vi "Camera.CaptureImage.vi"(8 "error in (no error)":errorcluster, 11 "Camera.Simulated":refnum<class "Camera.Simulated.lvclass">) -> (0 "error out":errorcluster, 2 "buffer":i32, 3 "Camera.Simulated out":refnum<class "Camera.Simulated.lvclass">)   [LabVIEW 2013, in "Camera.Simulated.lvclass"]
doc: "---------------------------------------------------------------\nJKI State Machine Objects™\nhttp://jki.net/state-machine-objects/\nCopyright (C) 2005-2015, JKI <info@jki.net>\nALL RIGHTS RESERVEDJKI State Machine Objects (SMO) 1.0.0.5\nJKI - JKI\nCopyright (c) 2016, JKI"
uses:
  Camera.Simulated.lvclass
  CircularBuffer/CircularBuffer.lvclass
  CircularBuffer.ImageData/CircularBuffer.ImageData.lvclass
  Camera/Camera.lvclass
panel:
  # "For instructions on how to use the JKI State Machine Objects, examples and video tutorials, visit:\nhttp://jki.net/state-machine-objects/\n\nJKI State Machine Objects™\nhttp://jki.net/state-machine-objects/\nCopyright (C) 2005-2015, JKI <info@jki.net>\nALL RIGHTS RESERVED"
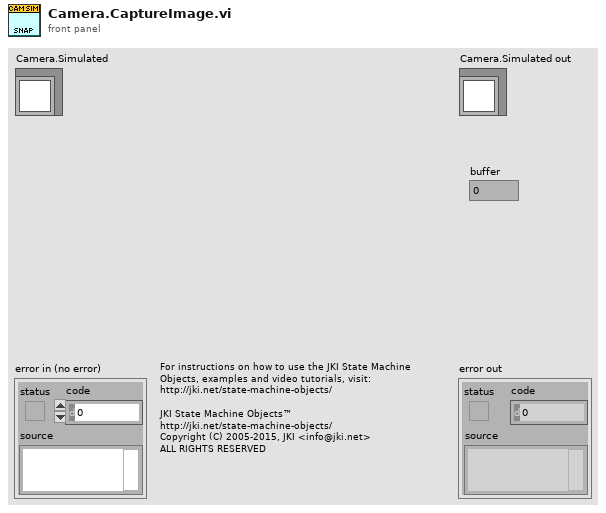
[diagram p1: front panel]
types:
  T1 = typedef "Camera.Simulated.lvclass/Dependencies--Cluster.ctl" = cluster{"CircularBuffer.ImageData":refnum<class "CircularBuffer.ImageData.lvclass">}
  T2 = typedef "imagedata.ctl" = cluster{"image type":i32, "image depth":i32, "image":u8[], "mask":u8[], "colors":u32[], "Rectangle":cluster{"left":i16, "top":i16, "right":i16, "bottom":i16}}
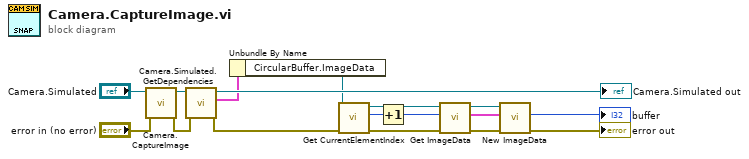
[diagram p0: block diagram]
diagram:
  n1 = call-parent "Camera.CaptureImage.vi"("error in (no error)"="error in (no error)", "Camera"="Camera.Simulated") -> ("error out"=w14:errorcluster, "Camera out"=w16:refnum<class "Camera.Simulated.lvclass">)  [unwired: 7 in, 1 out]
  n2 = call "Camera.Simulated.GetDependencies.vi"("error in (no error)"=w14, "Camera.Simulated"=w16) -> ("error out"=w11:errorcluster, "Dependencies"=w12:T1, "Camera.Simulated"=→"Camera.Simulated out":refnum<class "Camera.Simulated.lvclass">)  [unwired: 7 in]
  n3 = Unbundle By Name(w12) -> ("CircularBuffer.ImageData"=w9:refnum<class "CircularBuffer.ImageData.lvclass">)
  n4 = call "Get CurrentElementIndex.vi"("error in (no error)"=w11, "CircularBuffer"=w9) -> ("error out"=w3:errorcluster, "Current Element index"=w10:i32, "CircularBuffer out"=w1:refnum<class "CircularBuffer.ImageData.lvclass">)  [unwired: 7 in]
  n5 = Increment(x=w10) -> (x+1=w6:i32)
  n6 = call "Get ImageData.vi"("error in (no error)"=w3, "GetElement (-1: Current)"=w6, "CircularBuffer.ImageData"=w1) -> ("error out"=w4:errorcluster, "ImageData"=w7:T2, "CircularBuffer.ImageData out"=w8:refnum<class "CircularBuffer.ImageData.lvclass">)  [unwired: 6 in]
  n7 = call "New ImageData.vi"("error in (no error)"=w4, "ImageData"=w7, "CircularBuffer.ImageData"=w8) -> ("error out"=→"error out":errorcluster, "newElementIndex"=→"buffer":i32)  [unwired: 6 in, 1 out]
